vi "FTMS_beta.vi"() -> ()   [LabVIEW 2011]
doc: "Enables and disables RF output of PSG1 & PSG2"
uses:
  Hardware Control/OSC/SubVIs/controls/sampling_rate.ctl
  Hardware Control/OSC/SubVIs/controls/scale.ctl
  global.vi
panel:
  out "waiting":bool
  in  "Pause":bool
  in  "Stop":bool
  out "current step":i32
  out "current frequency":dbl format="%6.2p"
  out "current meas cycle":i32
  out "dt":dbl format="%#_6p"
  out "reset meas cycle timer":bool
  out "first start":bool
  in  "Tab Control":T1(tab)
  in  "EXP Meas Period (s)":dbl=10.0 min=1.0 format="%.2g"
  in  "Purge Freq.":dbl=2.0 caption="Purge Freq. (Hz)"
  in  "PURGE nozzle":bool
  in  "Refresh meas time":bool
  out "meas cycle time (ms)":u32
  in  "start experiment":bool
  in  "config TRIG":bool
  in  "config OSC":bool
  out "OSC resolution":ext=24999.999999999999998 caption="Resolution (Hz)" format="%#_6p"
  out "OSC sample points":i32=200000 caption="points / frame"
  out "TRIG BG cycle":dbl=100.0 caption="BG. cycle" min=0.0 max=999.999999999995 format="%.2p"
  out "TRIG mol delay":dbl=9.999999999999999e-05 caption="Mol. delay" min=0.0 max=999.999999999995 format="%.2p"
  out "TRIG start time":dbl[](array[numeric])=[0.0, 1.1e-06, 6.6e-06, 6.4e-06] caption="delay starts (s)" format="%.3p"
  out "TRIG burst enable":bool=TRUE caption="Burst"
  out "TRIG delay duration":dbl=4.6625e-05 caption="delay cycle (s)" format="%.2p"
  out "TRIG duration":dbl[](array[numeric])=[5.65e-06, 4.9999999999999996e-06, 4e-05, 4.9999999999999996e-06] caption="delay durations (s)" min=0.0 format="%.3p"
  out "TRIG burst period":dbl=4.9999999999999975e-05 caption="burst period (s)" format="%.2p"
  out "TRIG burst count":i32=1 caption="burst count"
  out "OSC hor scale":T2=4e-06 items=["400ns/div"=4e-07, "1µs/div"=1e-06, "2µs/div"=2e-06, "4µs/div"=4e-06, "10µs/div"=1e-05, "20µs/div"=2e-05]
  out "OSC sample rate":T3=5000000000.0 items=["20 GHz (50ps/sample)", "10 GHz (100ps/sample)", "5.0 GHz (200ps/sample)", "2.5 GHz (400ps/sample)", "1.25 GHz (0.8ns/sample)", "0.5 GHz (2ns/sample)"]
  in  "EXP Meas Cycles":i32=10 min=1 step=1
  in  "PSG start freq":dbl=0.0003 caption="Start Freq. (Hz)" min=0.00025 max=67.0 step=1e-06 format="%#.12p"
  in  "PSG Amplitude1":dbl caption="PSG1 Ampl (dBm)" min=-135.0 max=30.0 step=0.5 format="%#_8p"
  in  "PSG Amplitude 2":dbl caption="PSG2 Ampl (dBm)" min=-135.0 max=30.0 step=0.5 format="%#_8p"
  in  "PSG freq offset":dbl=0.0003 caption="freq. offset (Hz)" min=0.00025 max=67.0 step=1e-06 format="%#.12p"
  in  "write configs":bool
  in  "load config":bool
  in  "save config":bool
  in  "PSG steps":u32=1 min=1 step=1 format="%.0p"
  in  "PSG step size":dbl=0.0003 caption="step size" min=0.00025 max=67.0 step=1e-06 format="%#.12p"
  out "Meas Time":string="00:00:00"
  out "Experiment Time":string="00:00:00"
  in  "EXP chirp end":dbl=1000000000.0 format="%.2p"
  out "meas duration":dbl format="%.1p"
  out "Current Molecular Frame":T4(graph) caption="Molecular Frame"
  out "Current Background Frame":T4(graph) caption="Background Frame"
  out "Current Cor Spectra":T4(graph) caption="Corrected Frame"
  out "frame averages completed:":i32 caption="averages:"
  in  "Frame":i32=1 caption="Displayed Frame" min=1 step=1
  in  "reset frame average":bool
  in  "frame single cycle":bool caption="no averaging"
  out "Average Cor":T4(graph) caption="Average of all corrected time domain signals"
  out "Averaged Background":T4(graph)
  out "Averaged Molecular":T4(graph)
  in  "Quit":bool
  # "local variables"
  # "General Settings"
  # "PSG Configuration"
  # "TRIG Configuration"
  # "OSC Configuration"
  # "File Storage"
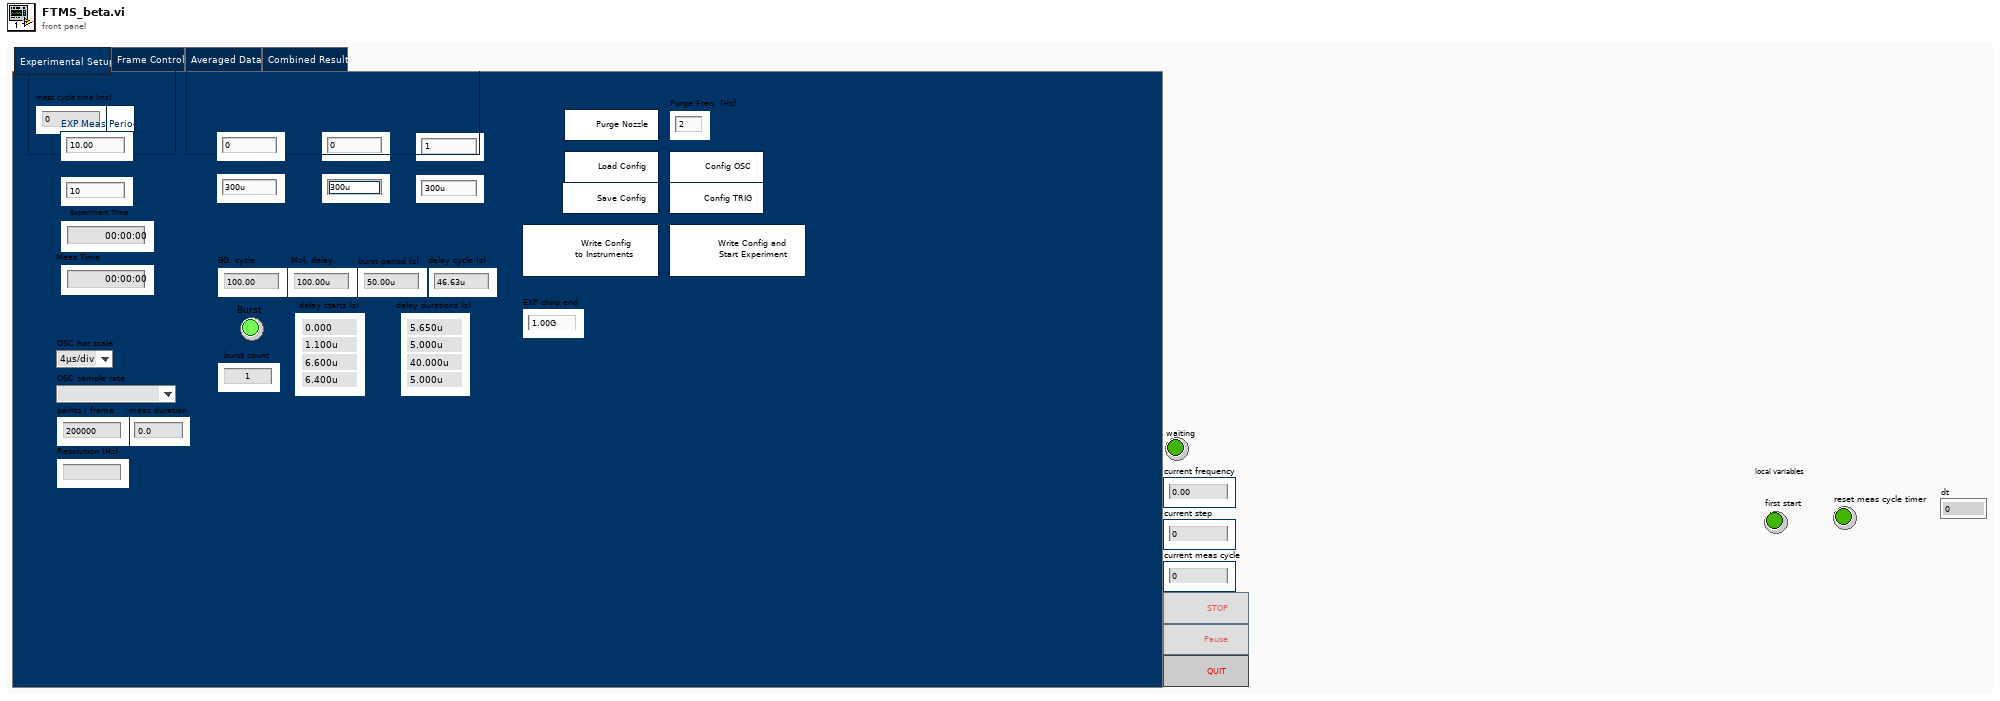
[diagram p1: front panel]
types:
  T1 = enum32{"Experimental Setup", "Frame Control", "Averaged Data", "Combined Result"}
  T2 = typedef "scale.ctl" = dbl
  T3 = typedef "sampling_rate.ctl" = ext
  T4 = cluster{"Numeric Control":dbl, "df":dbl, "magnitude":dbl[]}
  T5 = enum8{"Enabled", "Disabled", "Disabled and Grayed Out"}
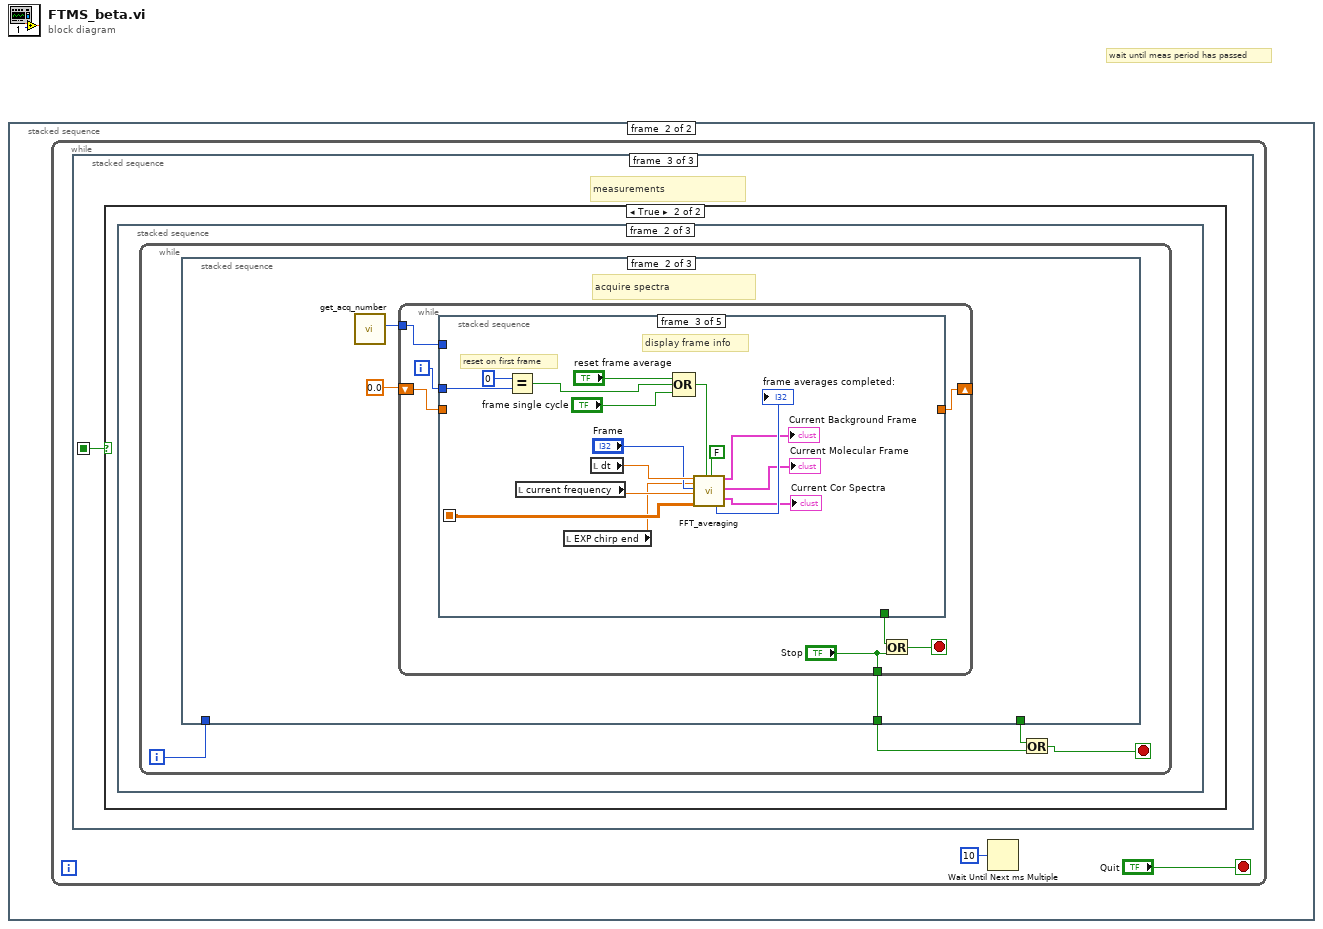
[diagram p0: block diagram]
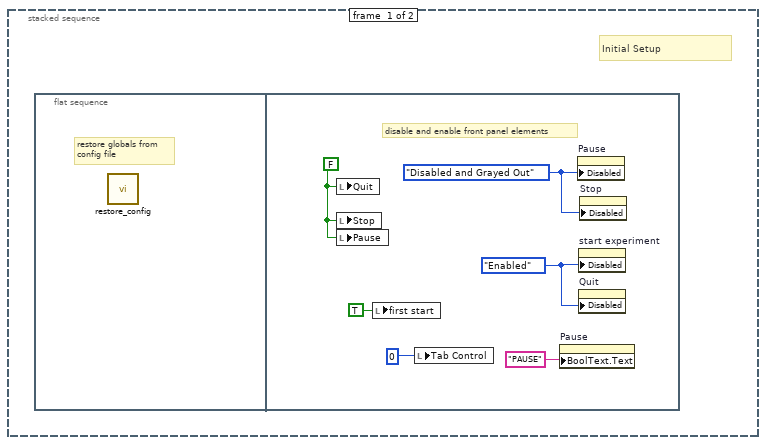
[diagram p2: hidden frame]
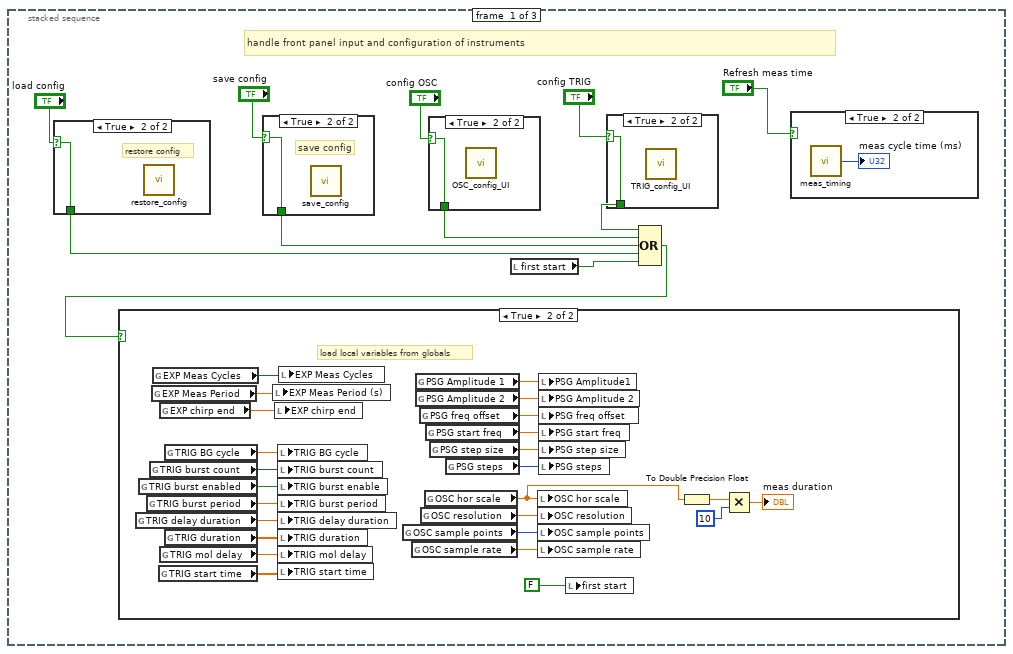
[diagram p3: hidden frame]
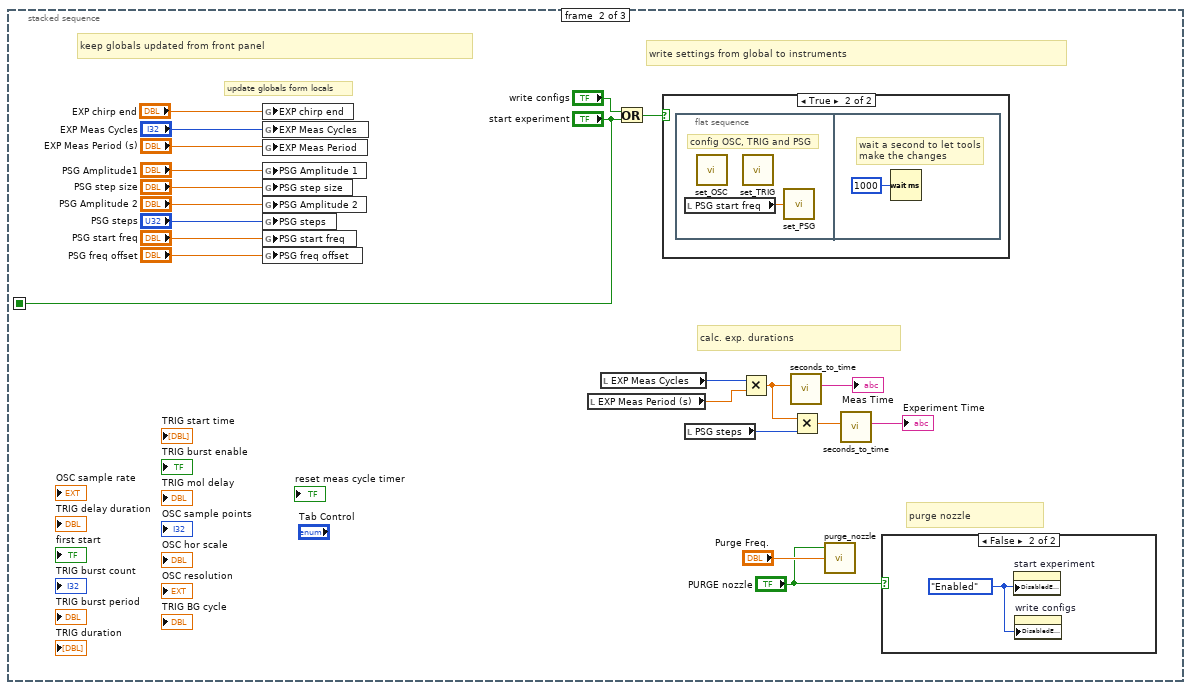
[diagram p10: hidden frame]
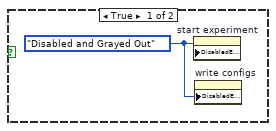
[diagram p11: hidden frame]
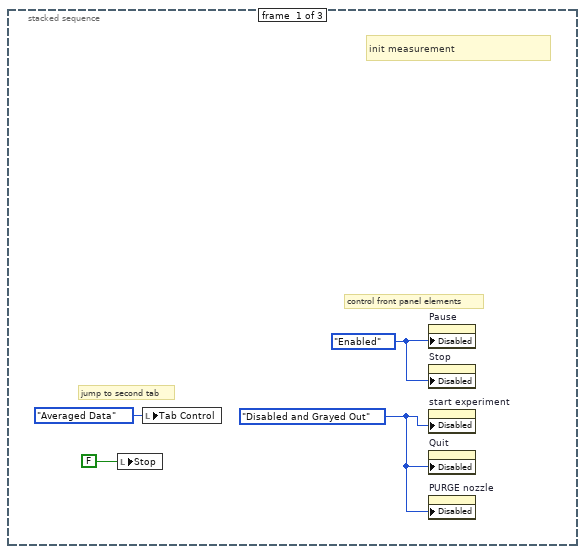
[diagram p14: hidden frame]
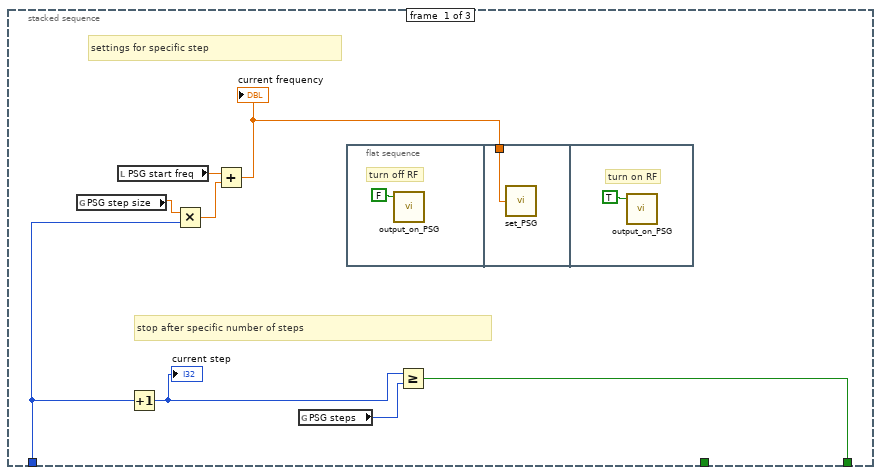
[diagram p15: hidden frame]
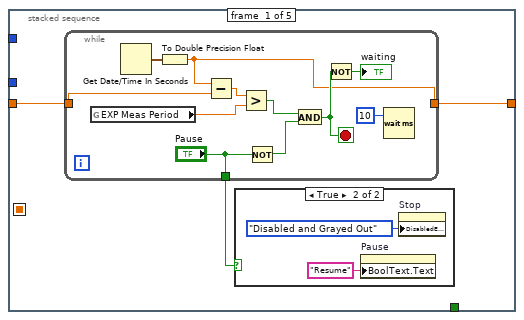
[diagram p16: hidden frame]
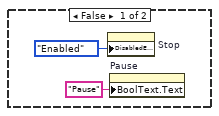
[diagram p17: hidden frame]
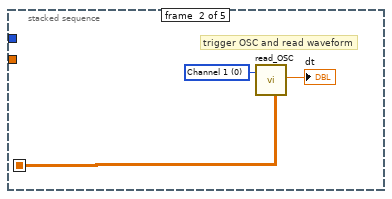
[diagram p18: hidden frame]
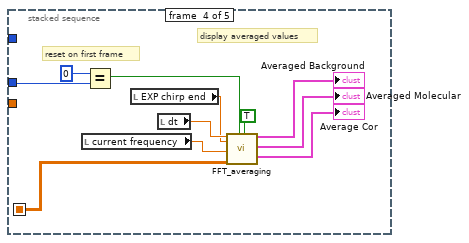
[diagram p19: hidden frame]
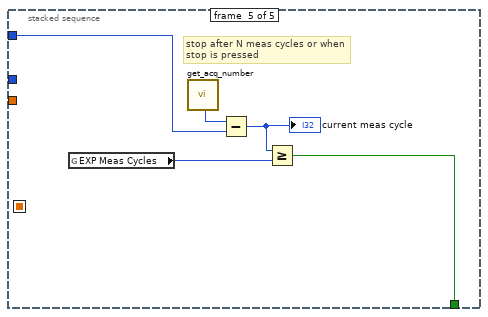
[diagram p20: hidden frame]
diagram:
  # "wait until meas period has passed"
  n1 = stacked-sequence {
    frame #0 {
      # "Initial Setup"
      n2 = flat-sequence {
        frame #0 {
          # "restore globals from\nconfig file"
          n3 = call "restore_config.vi"() -> ()  [unwired: 5 in]
        }
        frame #1 {
          w5 = T5."Disabled and Grayed Out" ("Disabled")
          w2 = T5."Enabled" ("Disabled")
          w6 = FALSE ("Quit")
          # "disable and enable front panel elements"
          n4 = local write "Quit"(w6) -> ()
          n5 = local write "Stop"(w6) -> ()
          n6 = local write "Pause"(w6) -> ()
          n7 = local write "first start"(TRUE ("first start")) -> ()
          n8 = local write "Tab Control"(0) -> ()
          n9 = property on="Pause" class="Bool (strict)"("BoolText.Text"="PAUSE" ("Boolean Text.Text")) -> ()  [unwired: 2 in, 2 out]
          n10 = property on="Pause" class="Bool (strict)"("Disabled"=w5) -> ()  [unwired: 2 in, 2 out]
          n11 = property on="start experiment" class="Bool"("Disabled"=w2) -> ()  [unwired: 2 in, 2 out]
          n12 = property on="Quit" class="Bool (strict)"("Disabled"=w2) -> ()  [unwired: 2 in, 2 out]
          n13 = property on="Stop" class="Bool (strict)"("Disabled"=w5) -> ()  [unwired: 2 in, 2 out]
        }
      }
    }
    frame #1 {
      n14 = while {
        stop <- "Quit" stop-if-true
        n15 = stacked-sequence {
          seq-local: [_ "start experiment" _] -> [_ _ w79]
          frame #0 {
            # "handle front panel input and configuration of instruments"
            n16 = case shown="True" "load config" {
              selector: "load config" -> [w52 w53]
              tunnel: [w52 w53] -> w11
              frame False {
              }
              frame True {
                # "restore config"
                n17 = call "restore_config.vi"() -> ()  [unwired: 5 in]
              }
            }
            n18 = case shown="True" "save config" {
              selector: "save config" -> [w50 w51]
              tunnel: [w50 w51] -> w13
              frame False {
              }
              frame True {
                # "save config"
                n19 = call "save_config.vi"() -> ()  [unwired: 5 in]
              }
            }
            n20 = case shown="True" "config OSC" {
              selector: "config OSC" -> [w48 w49]
              tunnel: [w48 w49] -> w15
              frame False {
              }
              frame True {
                n21 = call "OSC_config_UI.vi"() -> ()  [unwired: 12 in]
              }
            }
            n22 = local read "first start"() -> (w18:bool)
            n23 = case shown="True" "config TRIG" {
              selector: "config TRIG" -> [w46 w47]
              tunnel: [w46 w47] -> w16
              frame False {
              }
              frame True {
                n24 = call "TRIG_config_UI.vi"() -> ()  [unwired: 12 in]
              }
            }
            n25 = Compound Arithmetic op=OR(w16, w15, w13, w11, w18) -> (w10:bool)
            n26 = case shown="True" w10 {
              frame False {
              }
              frame True {
                # "load local variables from globals"
                n27 = global read "global.vi" "TRIG delay duration"() -> (w31:dbl)
                n28 = global read "global.vi" "TRIG burst enabled"() -> (w33:bool)
                n29 = global read "global.vi" "TRIG burst period"() -> (w32:dbl)
                n30 = global read "global.vi" "TRIG burst count"() -> (w34:i32)
                n31 = global read "global.vi" "EXP Meas Period"() -> (w26:dbl)
                n32 = global read "global.vi" "EXP Meas Cycles"() -> (w45:i32)
                n33 = global read "global.vi" "TRIG start time"() -> (w28:dbl[])
                n34 = global read "global.vi" "EXP chirp end"() -> (w21:dbl)
                n35 = global read "global.vi" "TRIG mol delay"() -> (w29:dbl)
                n36 = global read "global.vi" "TRIG BG cycle"() -> (w35:dbl)
                n37 = global read "global.vi" "TRIG duration"() -> (w30:dbl[])
                n38 = local write "EXP Meas Period (s)"(w26) -> ()
                n39 = local write "EXP chirp end"(w21) -> ()
                n40 = local write "TRIG BG cycle"(w35) -> ()
                n41 = local write "TRIG burst count"(w34) -> ()
                n42 = local write "TRIG burst enable"(w33) -> ()
                n43 = local write "TRIG burst period"(w32) -> ()
                n44 = local write "TRIG delay duration"(w31) -> ()
                n45 = local write "TRIG duration"(w30) -> ()
                n46 = local write "TRIG mol delay"(w29) -> ()
                n47 = local write "TRIG start time"(w28) -> ()
                n48 = local write "EXP Meas Cycles"(w45) -> ()
                n49 = global read "global.vi" "OSC sample points"() -> (w43:i32)
                n50 = global read "global.vi" "OSC sample rate"() -> (w42:T3)
                n51 = global read "global.vi" "PSG Amplitude 1"() -> (w37:dbl)
                n52 = global read "global.vi" "PSG Amplitude 2"() -> (w38:dbl)
                n53 = global read "global.vi" "PSG freq offset"() -> (w39:dbl)
                n54 = global read "global.vi" "OSC resolution"() -> (w44:ext)
                n55 = global read "global.vi" "OSC hor scale"() -> (w22:T2)
                n56 = global read "global.vi" "PSG start freq"() -> (w40:dbl)
                n57 = global read "global.vi" "PSG step size"() -> (w41:dbl)
                n58 = global read "global.vi" "PSG steps"() -> (w36:i32)
                n59 = local write "OSC hor scale"(w22) -> ()
                n60 = local write "OSC resolution"(w44) -> ()
                n61 = local write "OSC sample points"(w43) -> ()
                n62 = local write "OSC sample rate"(w42) -> ()
                n63 = local write "PSG Amplitude1"(w37) -> ()
                n64 = local write "PSG Amplitude 2"(w38) -> ()
                n65 = local write "PSG freq offset"(w39) -> ()
                n66 = local write "PSG start freq"(w40) -> ()
                n67 = local write "PSG step size"(w41) -> ()
                n68 = local write "PSG steps"(w36) -> ()
                n69 = local write "first start"(FALSE ("first start")) -> ()
                n70 = To Double Precision Float(number=w22) -> (double precision float=w24:T2)
                n71 = Multiply(x=w24, y=10) -> (x*y=→"meas duration":T2)
              }
            }
            n72 = case shown="True" "Refresh meas time" {
              frame False {
              }
              frame True {
                n73 = call "meas_timing.vi"() -> ("meas cycle time"=→"meas cycle time (ms)":u32)  [unwired: 5 in]
              }
            }
          }
          frame #1 {
            # "calc. exp. durations"
            # "purge nozzle"
            # "write settings from global to instruments"
            # "keep globals updated from front panel"
            # "update globals form locals"
            n74 = global write "global.vi" "EXP chirp end"("EXP chirp end") -> ()
            n75 = global write "global.vi" "EXP Meas Cycles"("EXP Meas Cycles") -> ()
            n76 = global write "global.vi" "EXP Meas Period"("EXP Meas Period (s)") -> ()
            n77 = global write "global.vi" "PSG Amplitude 1"("PSG Amplitude1") -> ()
            n78 = global write "global.vi" "PSG step size"("PSG step size") -> ()
            n79 = global write "global.vi" "PSG Amplitude 2"("PSG Amplitude 2") -> ()
            n80 = global write "global.vi" "PSG steps"("PSG steps") -> ()
            n81 = global write "global.vi" "PSG start freq"("PSG start freq") -> ()
            n82 = global write "global.vi" "PSG freq offset"("PSG freq offset") -> ()
            n83 = local read "EXP Meas Period (s)"() -> (w61:dbl)
            n84 = local read "EXP Meas Cycles"() -> (w62:i32)
            n85 = Or(x="write configs", y="start experiment") -> (x .or. y?=w66:bool)
            n86 = case shown="True" w66 {
              frame False {
              }
              frame True {
                n87 = flat-sequence {
                  frame #0 {
                    # "config OSC, TRIG and PSG"
                    n88 = local read "PSG start freq"() -> (w77:dbl)
                    n89 = call "set_OSC.vi"() -> ()  [unwired: 12 in]
                    n90 = call "set_TRIG.vi"() -> ()  [unwired: 12 in]
                    n91 = call "set_PSG.vi"("PSG1 frequency"=w77) -> ()  [unwired: 5 in]
                  }
                  frame #1 {
                    # "wait a second to let tools \nmake the changes"
                    n92 = Wait (ms)(milliseconds to wait=u32 1000) -> ()  [unwired: 1 out]
                  }
                }
              }
            }
            n93 = local read "PSG steps"() -> (w58:u32)
            n94 = Multiply(x=w62, y=w61) -> (x*y=w59:dbl)
            n95 = call "seconds_to_time.vi"("# Seconds (0)"=w59) -> ("Elapsed Time (00:00:00)"=→"Meas Time":string)  [unwired: 10 in]
            n96 = Multiply(x=w59, y=w58) -> (x*y=w56:dbl)
            n97 = call "purge_nozzle.vi"("purge frequency"="Purge Freq.", "Purge"="PURGE nozzle") -> ()  [unwired: 4 in]
            n98 = call "seconds_to_time.vi"("# Seconds (0)"=w56) -> ("Elapsed Time (00:00:00)"=→"Experiment Time":string)  [unwired: 10 in]
            n99 = case shown="False" "PURGE nozzle" {
              frame True {
                w75 = T5."Disabled and Grayed Out" ("Disabled")
                n100 = property on="start experiment" class="Bool"("DisabledEnum"=w75) -> ()  [unwired: 2 in, 2 out]
                n101 = property on="write configs" class="Bool"("DisabledEnum"=w75) -> ()  [unwired: 2 in, 2 out]
              }
              frame False {
                w76 = T5."Enabled" ("Disabled")
                n102 = property on="start experiment" class="Bool"("DisabledEnum"=w76) -> ()  [unwired: 2 in, 2 out]
                n103 = property on="write configs" class="Bool"("DisabledEnum"=w76) -> ()  [unwired: 2 in, 2 out]
              }
            }
          }
          frame #2 {
            # "measurements"
            n104 = case shown="True" w79 {
              frame False {
              }
              frame True {
                n105 = stacked-sequence {
                  frame #0 {
                    w83 = T5."Enabled" ("Disabled")
                    w82 = T5."Disabled and Grayed Out" ("Disabled")
                    # "init measurement"
                    # "control front panel elements"
                    # "jump to second tab"
                    n106 = local write "Stop"(FALSE ("Stop")) -> ()
                    n107 = local write "Tab Control"(T1."Averaged Data" ("Tab Control")) -> ()
                    n108 = property on="Pause" class="Bool (strict)"("Disabled"=w83) -> ()  [unwired: 2 in, 2 out]
                    n109 = property on="Stop" class="Bool (strict)"("Disabled"=w83) -> ()  [unwired: 2 in, 2 out]
                    n110 = property on="start experiment" class="Bool"("Disabled"=w82) -> ()  [unwired: 2 in, 2 out]
                    n111 = property on="Quit" class="Bool (strict)"("Disabled"=w82) -> ()  [unwired: 2 in, 2 out]
                    n112 = property on="PURGE nozzle" class="Bool (strict)"("Disabled"=w82) -> ()  [unwired: 2 in, 2 out]
                  }
                  frame #1 {
                    n113 = while {
                      i -> [w87]
                      stop <- w85 stop-if-true
                      n114 = stacked-sequence {
                        tunnel: w87 -> [w92 _ _]
                        tunnel: [w91 _ _] -> w86
                        tunnel: [_ w99 _] -> w84
                        frame #0 {
                          # "stop after specific number of steps"
                          # "settings for specific step"
                          n115 = global read "global.vi" "PSG step size"() -> (w95:dbl)
                          n116 = local read "PSG start freq"() -> (w94:dbl)
                          n117 = Increment(x=w92) -> (x+1=w89:i32)
                          "current step" <- w89
                          n118 = Multiply(x=w95, y=w92) -> (x*y=w93:dbl)
                          n119 = Add(x=w94, y=w93) -> (x+y=w88:dbl)
                          "current frequency" <- w88
                          n120 = global read "global.vi" "PSG steps"() -> (w90:i32)
                          n121 = flat-sequence {
                            tunnel: w88 -> [w97]
                            frame #0 {
                              # "turn off RF"
                              n122 = call "output_on_PSG.vi"("Enable RF Output (F:Disable)"=FALSE) -> ()  [unwired: 5 in]
                            }
                            frame #1 {
                              n123 = call "set_PSG.vi"("PSG1 frequency"=w97) -> ()  [unwired: 5 in]
                            }
                            frame #2 {
                              # "turn on RF"
                              n124 = call "output_on_PSG.vi"("Enable RF Output (F:Disable)"=TRUE) -> ()  [unwired: 5 in]
                            }
                          }
                          n125 = Greater Or Equal?(x=w89, y=w90) -> (x >= y?=w91:bool)
                        }
                        frame #1 {
                          # "acquire spectra"
                          n126 = call "get_acq_number.vi"() -> ("# of meas cycles"=w100:i32)  [unwired: 8 in, 3 out]
                          n127 = while {
                            tunnel: w100 -> [w107]
                            shift-right: [w105] -> _
                            shift-left: 0.0 -> [w104]
                            tunnel: ["Stop"] -> w99
                            i -> [w108]
                            stop <- w103 stop-if-true
                            n128 = stacked-sequence {
                              seq-local: [_ w129 _ _ _] -> [_ _ w138 w150 _]
                              tunnel: w108 -> [_ _ w140 w154 _]
                              tunnel: w107 -> [_ _ _ _ w160]
                              tunnel: [_ _ _ _ w159] -> w106
                              tunnel: [w111 _ _ _ _] -> w105
                              tunnel: w104 -> [w110 _ _ _ _]
                              frame #0 {
                                n129 = while {
                                tunnel: [w119] -> w111
                                tunnel: w110 -> [w125]
                                tunnel: ["Pause"] -> w109
                                stop <- w121 stop-if-true
                                n130 = global read "global.vi" "EXP Meas Period"() -> (w123:dbl)
                                n131 = Get Date/Time In Seconds() -> (seconds since 1Jan1904=w126:timestamp)
                                n132 = To Double Precision Float(number=w126) -> (double precision float=w119:dbl)
                                n133 = Subtract(x=w119, y=w125) -> (x-y=w124:dbl)
                                n134 = Greater?(x=w124, y=w123) -> (0:w118:bool)
                                n135 = Not(x="Pause") -> (.not. x?=w117:bool)
                                n136 = And(x=w118, y=w117) -> (x .and. y?=w121:bool)
                                n137 = Not(x=w121) -> (.not. x?=→"waiting":bool)
                                n138 = Wait (ms)(milliseconds to wait=u32 10) -> ()  [unwired: 1 out]
                                }
                                n139 = case shown="True" w109 {
                                frame False {
                                n140 = property on="Stop" class="Bool (strict)"("DisabledEnum"=T5."Enabled" ("Disabled")) -> ()  [unwired: 2 in, 2 out]
                                n141 = property on="Pause" class="Bool (strict)"("BoolText.Text"="Pause" ("Caption.Text")) -> ()  [unwired: 2 in, 2 out]
                                }
                                frame True {
                                n142 = property on="Pause" class="Bool (strict)"("BoolText.Text"="Resume" ("Caption.Text")) -> ()  [unwired: 2 in, 2 out]
                                n143 = property on="Stop" class="Bool (strict)"("DisabledEnum"=T5."Disabled and Grayed Out" ("Disabled")) -> ()  [unwired: 2 in, 2 out]
                                }
                                }
                              }
                              frame #1 {
                                w128 = u16 0 items=["Channel 1", "Channel 2", "Channel 3", "Channel 4", "Math 1", "Math 2", "Math 3", "Math 4", "Reference 1", "Reference 2", "Reference 3", "Reference 4"] ("Channel (0: Channel 1)")
                                # "trigger OSC and read waveform"
                                n144 = call "read_OSC.vi"("Channel (0: Channel 1)"=w128) -> ("appended array"=w129:dbl[][][], "dt"=→"dt":dbl)  [unwired: 7 in, 2 out]
                              }
                              frame #2 {
                                # "reset on first frame"
                                # "display frame info"
                                n145 = Equal?(x=0, y=w140) -> (x = y?=w136:bool)
                                n146 = local read "current frequency"() -> (w144:dbl)
                                n147 = local read "EXP chirp end"() -> (w130:dbl)
                                n148 = local read "dt"() -> (w145:dbl)
                                n149 = Compound Arithmetic op=OR("reset frame average", w136, "frame single cycle") -> (w134:bool)
                                n150 = call "FFT_averaging.vi"("dt"=w145, "chirp end"=w130, "frame"="Frame", "current frequency"=w144, "3d waveform array"=w138, "reset frame average"=w134, "all frames?"=FALSE) -> ("averages compl"=→"frame averages completed:":i32, "BG spectrum"=→"Current Background Frame":T4, "Mol spectrum"=→"Current Molecular Frame":T4, "cor spectrum"=→"Current Cor Spectra":T4)  [unwired: 6 in, 3 out]
                              }
                              frame #3 {
                                # "reset on first frame"
                                # "display averaged values"
                                n151 = local read "current frequency"() -> (w152:dbl)
                                n152 = Equal?(x=0, y=w154) -> (x = y?=w151:bool)
                                n153 = local read "EXP chirp end"() -> (w147:dbl)
                                n154 = local read "dt"() -> (w153:dbl)
                                n155 = call "FFT_averaging.vi"("dt"=w153, "chirp end"=w147, "current frequency"=w152, "3d waveform array"=w150, "reset frame average"=w151, "all frames?"=TRUE) -> ("BG spectrum"=→"Averaged Background":T4, "Mol spectrum"=→"Averaged Molecular":T4, "cor spectrum"=→"Average Cor":T4)  [unwired: 7 in, 4 out]
                              }
                              frame #4 {
                                # "stop after N meas cycles or when \nstop is pressed"
                                n156 = global read "global.vi" "EXP Meas Cycles"() -> (w157:i32)
                                n157 = call "get_acq_number.vi"() -> ("# of meas cycles"=w161:i32)  [unwired: 8 in, 3 out]
                                n158 = Subtract(x=w161, y=w160) -> (x-y=w158:i32)
                                "current meas cycle" <- w158
                                n159 = Greater Or Equal?(x=w158, y=w157) -> (x >= y?=w159:bool)
                              }
                            }
                            n160 = Or(x=w106, y="Stop") -> (x .or. y?=w103:bool)
                          }
                        }
                        frame #2 {
                          # "save between steps as backup, overwrite old files"
                        }
                      }
                      n161 = Or(x=w86, y=w84) -> (x .or. y?=w85:bool)
                    }
                  }
                  frame #2 {
                    w165 = T5."Disabled and Grayed Out" ("Disabled")
                    w164 = T5."Enabled" ("Disabled")
                    # "turn off RF"
                    n162 = local write "Stop"(FALSE ("Stop")) -> ()
                    n163 = call "output_on_PSG.vi"("Enable RF Output (F:Disable)"=FALSE) -> ()  [unwired: 5 in]
                    n164 = property on="Pause" class="Bool (strict)"("Disabled"=w165) -> ()  [unwired: 2 in, 2 out]
                    n165 = property on="Stop" class="Bool (strict)"("Disabled"=w165) -> ()  [unwired: 2 in, 2 out]
                    n166 = property on="start experiment" class="Bool"("Disabled"=w164) -> ()  [unwired: 2 in, 2 out]
                    n167 = property on="Quit" class="Bool (strict)"("Disabled"=w164) -> ()  [unwired: 2 in, 2 out]
                    n168 = property on="PURGE nozzle" class="Bool (strict)"("Disabled"=w164) -> ()  [unwired: 2 in, 2 out]
                  }
                }
              }
            }
          }
        }
        n169 = Wait Until Next ms Multiple(millisecond multiple=u32 10) -> ()  [unwired: 1 out]
      }
    }
  }
